vi "Triangle Demo Init Solution.vi"() -> (3 "shape array":refnum<class "Shape.lvclass">[](array[class]))   [LabVIEW 2015]
uses:
  Shape/Shape.lvclass
  Circle/Circle.lvclass
  Square/Square.lvclass
  colors.ctl
  Solution Triangle/Solution Triangle.lvclass
  Circle/Circle.lvclass/Circle.ctl
  Shape/Shape.lvclass/Shape.ctl
  Square/Square.lvclass/Square.ctl
  Solution Triangle/Solution Triangle.lvclass/Solution Triangle.ctl
  Solution Triangle/Write base.vi
  Solution Triangle/Write Height.vi
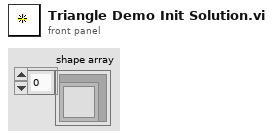
[diagram p1: front panel]
types:
  T1 = typedef "colors.ctl" = enum16{"Blue", "Red", "Green", "Yellow"}
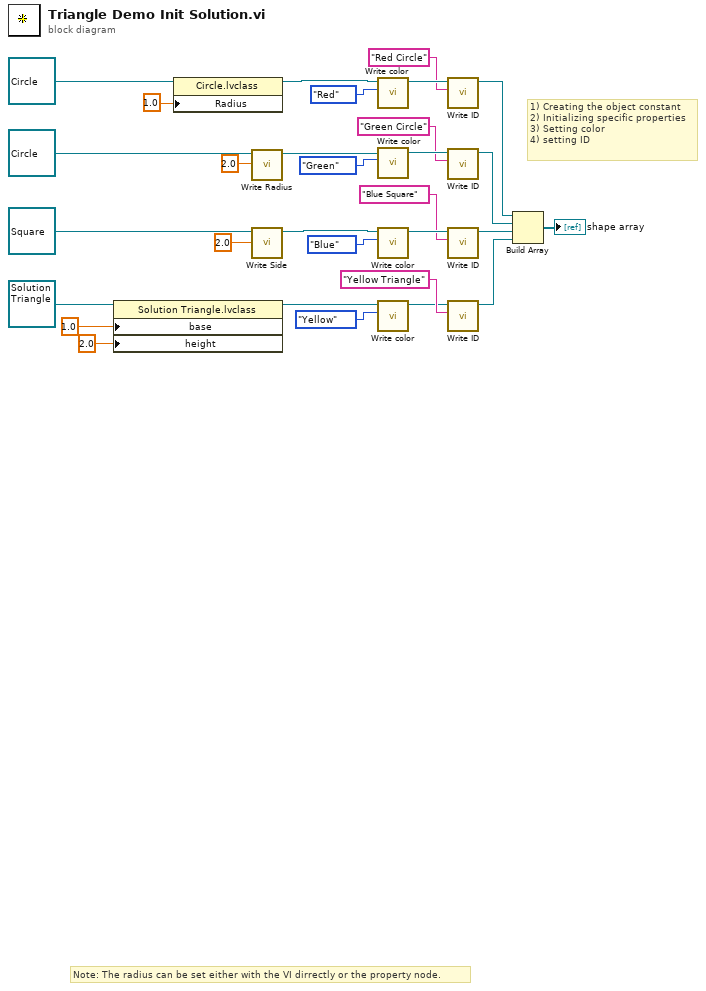
[diagram p0: block diagram]
diagram:
  # "1) Creating the object constant\n2) Initializing specific properties\n3) Setting color\n4) setting ID"
  # "Note: The radius can be set either with the VI dirrectly or the property node."
  n1 = property class="Solution Triangle.lvclass"(reference=refnum<class "Solution Triangle.lvclass"> refnum ("Solution Triangle.lvclass"), "base"=1.0, "height  "=2.0 ("height")) -> (reference out=w5:refnum<class "Solution Triangle.lvclass">)  [unwired: 1 in, 1 out]
  n2 = property class="Circle.lvclass"(reference=refnum<class "Circle.lvclass"> refnum ("Circle.lvclass"), "Radius"=1.0) -> (reference out=w28:refnum<class "Circle.lvclass">)  [unwired: 1 in, 1 out]
  n3 = call "Write Radius.vi"("Radius"=2.0, "Circle in"=refnum<class "Circle.lvclass"> refnum ("Circle.lvclass")) -> ("Circle out"=w12:refnum<class "Circle.lvclass">)  [unwired: 8 in, 1 out]
  n4 = call "Write Side.vi"("Side"=2.0, "Square in"=refnum<class "Square.lvclass"> refnum ("Square.lvclass")) -> ("Square out"=w22:refnum<class "Square.lvclass">)  [unwired: 8 in, 1 out]
  n5 = call "Write color.vi"("color"=colors."Red", "Shape in"=w28) -> ("Shape out"=w30:refnum<class "Circle.lvclass">)  [unwired: 8 in, 1 out]
  n6 = call "Write color.vi"("color"=colors."Green", "Shape in"=w12) -> ("Shape out"=w25:refnum<class "Circle.lvclass">)  [unwired: 8 in, 1 out]
  n7 = call "Write color.vi"("color"=colors."Blue", "Shape in"=w22) -> ("Shape out"=w23:refnum<class "Square.lvclass">)  [unwired: 8 in, 1 out]
  n8 = call "Write color.vi"("color"=colors."Yellow", "Shape in"=w5) -> ("Shape out"=w6:refnum<class "Solution Triangle.lvclass">)  [unwired: 8 in, 1 out]
  n9 = call "Write ID.vi"("ID"="Red Circle", "Shape in"=w30) -> ("Shape out"=w26:refnum<class "Circle.lvclass">)  [unwired: 8 in, 1 out]
  n10 = call "Write ID.vi"("ID"="Green Circle", "Shape in"=w25) -> ("Shape out"=w2:refnum<class "Circle.lvclass">)  [unwired: 8 in, 1 out]
  n11 = call "Write ID.vi"("ID"="Blue Square", "Shape in"=w23) -> ("Shape out"=w1:refnum<class "Square.lvclass">)  [unwired: 8 in, 1 out]
  n12 = call "Write ID.vi"("ID"="Yellow Triangle", "Shape in"=w6) -> ("Shape out"=w3:refnum<class "Solution Triangle.lvclass">)  [unwired: 8 in, 1 out]
  n13 = Build Array(w26, w2, w1, w3) -> (→"shape array":refnum<class "Shape.lvclass">[])
